vi "Write Base.vi"(8 "error in (no error)":errorcluster, 10 "Base":dbl, 11 "Rectangulo in":refnum<class "Rectangulo.lvclass">) -> (0 "error out":errorcluster, 3 "Rectangulo out":refnum<class "Rectangulo.lvclass">)   [LabVIEW 2024, in "Rectangulo.lvclass"]
uses:
  Rectangulo.lvclass
  Rectangulo.lvclass/Rectangulo.ctl
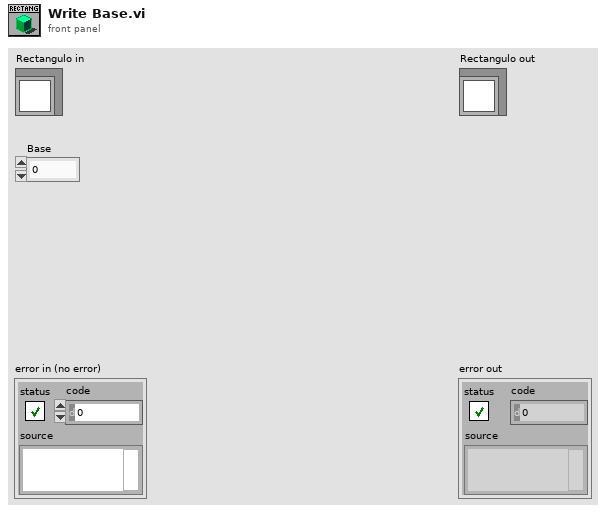
[diagram p1: front panel]
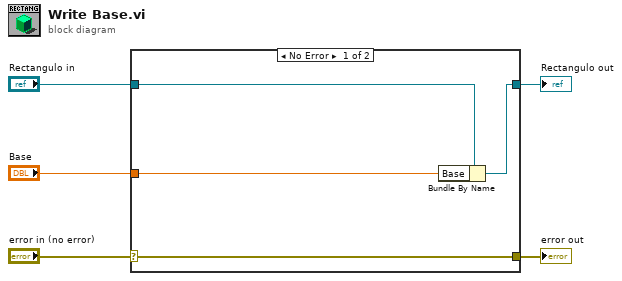
[diagram p0: block diagram]
diagram:
  n1 = case shown="No Error" "error in (no error)" {
    selector: "error in (no error)" -> [w9 w10]
    tunnel: [w9 w10] -> w4
    tunnel: [w7 w11] -> w2
    tunnel: "Rectangulo in" -> [w8 w11]
    tunnel: "Base" -> [w6 _]
    frame No Error {
      n2 = Bundle By Name(cluster=w8, "Base"=w6) -> (w7:refnum<class "Rectangulo.lvclass">)
    }
    frame Error {
    }
  }
  "error out" <- w4
  "Rectangulo out" <- w2
